vi "New Ball Stack.vi"(0 "Suck?":bool, 2 "spinOut?":bool, 3 "MiddleMS":T1, 4 "TopMS":T1, 5 "Top Stack Speed":dbl=0.5, 8 "CupMS":T1) -> (7 "Top":dbl, 9 "Middle":dbl, 10 "Floor":dbl)   [LabVIEW 2011]
uses:
  <vilib>/Rock Robotics/WPI/DigitalInput/WPI_DigitalInputDevRef.ctl
  <vilib>/Rock Robotics/SystemInterfaces/DIO/FPGA_DIOChannel.ctl
  <vilib>/Rock Robotics/SystemInterfaces/Typedef/FPGA_TypedefDigitalModule.ctl
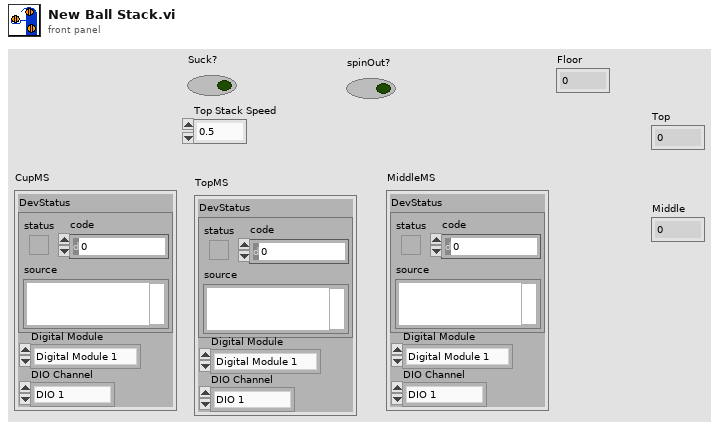
[diagram p1: front panel]
types:
  T1 = typedef "WPI_DigitalInputDevRef.ctl" = cluster{"DevStatus":errorcluster, "DIO Channel":T2, "Digital Module":T3}
  T2 = typedef "FPGA_DIOChannel.ctl" = enum8{"DIO 1", "DIO 2", "DIO 3", "DIO 4", "DIO 5", "DIO 6", "DIO 7", "DIO 8", "DIO 9", "DIO 10", "DIO 11", "DIO 12", "DIO 13", "DIO 14", "Invalid"}
  T3 = typedef "FPGA_TypedefDigitalModule.ctl" = enum16{"Digital Module 1", "Digital Module 2"}
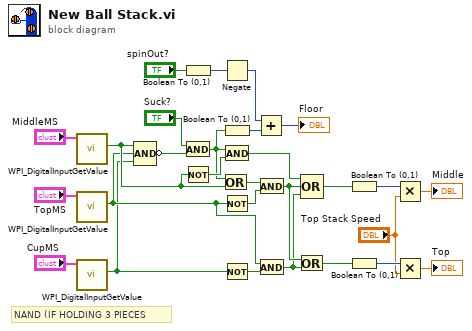
[diagram p0: block diagram]
diagram:
  # "NAND (IF HOLDING 3 PIECES"
  n1 = call <vilib>:"WPI_DigitalInputGetValue.vi"("DigitalInputDevRef"="MiddleMS") -> ("Value"=w5:bool)  [unwired: 8 in, 2 out]
  n2 = call <vilib>:"WPI_DigitalInputGetValue.vi"("DigitalInputDevRef"="TopMS") -> ("Value"=w3:bool)  [unwired: 8 in, 2 out]
  n3 = call <vilib>:"WPI_DigitalInputGetValue.vi"("DigitalInputDevRef"="CupMS") -> ("Value"=w1:bool)  [unwired: 8 in, 2 out]
  n4 = Compound Arithmetic op=AND(w5, w3, w1) -> (invert w9:bool)
  n5 = Boolean To (0,1)(Boolean="spinOut?") -> (0, 1=w27:i16)
  n6 = And(x="Suck?", y=w9) -> (x .and. y?=w8:bool)
  n7 = Not(x=w5) -> (.not. x?=w17:bool)
  n8 = Or(x=w8, y=w5) -> (x .or. y?=w23:bool)
  n9 = Negate(x=w27) -> (-x=w26:i16)
  n10 = Boolean To (0,1)(Boolean=w8) -> (0, 1=w25:i16)
  n11 = And(x=w8, y=w17) -> (x .and. y?=w16:bool)
  n12 = Not(x=w3) -> (.not. x?=w22:bool)
  n13 = Not(x=w1) -> (.not. x?=w21:bool)
  n14 = Add(x=w26, y=w25) -> (x+y=→"Floor":i16)
  n15 = And(x=w23, y=w22) -> (x .and. y?=w15:bool)
  n16 = And(x=w3, y=w21) -> (x .and. y?=w14:bool)
  n17 = Or(x=w15, y=w14) -> (x .or. y?=w20:bool)
  n18 = Compound Arithmetic op=OR(w16, w15, w14) -> (w11:bool)
  n19 = Boolean To (0,1)(Boolean=w11) -> (0, 1=w13:i16)
  n20 = Boolean To (0,1)(Boolean=w20) -> (0, 1=w19:i16)
  n21 = Multiply(x=w13, y="Top Stack Speed") -> (x*y=→"Middle":dbl)
  n22 = Multiply(x=w19, y="Top Stack Speed") -> (x*y=→"Top":dbl)
